vi "Teleop.vi"(10 "Match Info":T2={"Autonomous Elapsed Seconds"=0.0, "TeleOp Elapsed Seconds"=7.179, "Disabled Elapsed Seconds"=0.0, "Visited Autonomous"=FALSE, "Visited TeleOp"=TRUE, "Visited Disabled"=FALSE, "Autonomous Settings"={"Autonomous Style"=enum."Independent", "VI Refnum"=refnum}}, 11 "Call Context":T3=enum."Stop") -> ()   [LabVIEW 2020]
doc: "This VI is called for each TeleOp packet received from the DS where the robot is not disabled. It is often used to read from the joysticks and update I/O or to update setpoints for timed control loops. It should complete and return within 20 milliseconds or it may miss DS packets."
uses:
  <vilib>/Rock Robotics/WPI/DriverStation/WPI_DriverStationDerivedRobotMode.ctl
  <vilib>/Rock Robotics/WPI/DriverStation/WPI_DriverStationMatch Info.ctl
  <vilib>/Rock Robotics/WPI/ThirdParty/REV Robotics/REVLib/Typedef/Spark MAX Control Type.ctl
  <vilib>/Rock Robotics/WPI/ThirdParty/Sensors/navX/_TypeDefs/FRIC_navX_DeviceNumbersTypeDef.ctl
  <vilib>/Rock Robotics/WPI/ThirdParty/Phoenix-LabVIEW/CANCoder/Get/CTRE_Phoenix_CANcoder_GetSensorData.vi
  <vilib>/Rock Robotics/WPI/Utilities/WPI_GetSetVariantRefNum.vi
  <vilib>/addons/control/pid/pid.llb/PID (DBL).vi
  Robot Global Data.vi
  <vilib>/addons/control/pid/NI_PID_pid.lvlib
panel:
  in  "target angle":dbl=180.0
  out "MPUTemp":dbl=33.66
  in  "dt (s)":dbl=-1.0 format="%.3f"
  out "Yaw":dbl=-4.92
  in  "ScaleSpeed":dbl=0.5
  in  "PID gains 2":T1={"proportional gain (Kc)"=0.004667, "integral time (Ti, min)"=0.0, "derivative time (Td, min)"=0.0} {"derivative time (Td, min)" format="%.10f"; "integral time (Ti, min)" format="%.10f"; "proportional gain (Kc)" format="%.10f"}
  # "NOW WITH 200% MORE REV!!!!"
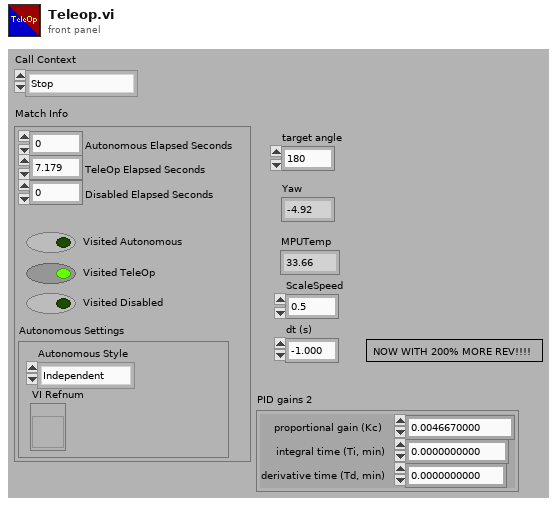
[diagram p1: front panel]
types:
  T1 = cluster{"proportional gain (Kc)":dbl, "integral time (Ti, min)":dbl, "derivative time (Td, min)":dbl}
  T2 = typedef "WPI_DriverStationMatch Info.ctl" = cluster{"Autonomous Elapsed Seconds":dbl, "TeleOp Elapsed Seconds":dbl, "Disabled Elapsed Seconds":dbl, "Visited Autonomous":bool, "Visited TeleOp":bool, "Visited Disabled":bool, "Autonomous Settings":cluster{"Autonomous Style":enum16{"Iterative", "Independent"}, "VI Refnum":refnum<vi>}}
  T3 = typedef "WPI_DriverStationDerivedRobotMode.ctl" = enum16{"Init", "Execute", "Stop"}
  T4 = typedef "FRIC_navX_DeviceNumbersTypeDef.ctl" = enum16{"Dev0", "Dev1", "Dev2", "Dev3"}
  T5 = typedef "Spark MAX Control Type.ctl" = enum16{"Percent VBus", "Voltage", "Velocity", "Position", "Smart Motion", "Current", "Smart Velocity"}
  T6 = typedef "WPI_JoystickDevRef.ctl" = cluster{"Device":T7}
  T7 = typedef "WPI_JoystickDeviceEnum.ctl" = enum16{"USB 0", "USB 1", "USB 2", "USB 3", "USB 4", "USB 5"}
  T8 = cluster{"Yaw":dbl, "Roll":dbl, "Pitch":dbl, "Heading":dbl, "Fused Heading":dbl}
  T9 = typedef "CTRE_Phoenix_CANcoder_DeviceRef.ctl" = cluster{"DeviceStatus":errorcluster, "Device Number":u8, "Handle":u64, "UsageFrame":u32, "Library Path":path}
  T10 = typedef "WPI_MotorControlDeviceRef.ctl" = cluster{"DeviceStatus":errorcluster, "Type":T11, "PWM":cluster{"PWM Channel":T12, "DeadBand":T13}, "CAN":cluster{"Device Number":u8, "SetOutput VI Ref":variant, "GetOutput VI Ref":variant, "Enable VI Ref":variant, "Disable VI Ref":variant, "Data":variant}, "Invert":bool, "DIO PWM":cluster{"PWM \"Enable\" Channel":T12, "DIOChannel":T14, "PWM Rate":dbl}}
  T11 = typedef "WPI_MotorControlType.ctl" = enum16{"PWM", "CAN", "DIO PWM"}
  T12 = typedef "FPGA_DIOPWMChannel.ctl" = enum8{"PWM 0", "PWM 1", "PWM 2", "PWM 3", "PWM 4", "PWM 5", "PWM 6", "PWM 7", "PWM 8", "PWM 9", "PWM MXP 0", "PWM MXP 1", "PWM MXP 2", "PWM MXP 3", "PWM MXP 4", "PWM MXP 5", "PWM MXP 6", "PWM MXP 7", "PWM MXP 8", "PWM MXP 9", "Invalid"}
  T13 = typedef "WPI_PWMDeadband.ctl" = cluster{"Name":string, "maxPositivePwm":i32, "minPositivePwm":i32, "centerPwm":i32, "maxNegativePwm":i32, "minNegativePwm":i32, "angularRange":u16}
  T14 = typedef "FPGA_DIOChannel.ctl" = enum8{"DIO 0", "DIO 1", "DIO 2", "DIO 3", "DIO 4", "DIO 5", "DIO 6", "DIO 7", "DIO 8", "DIO 9", "DIO MXP 0", "DIO MXP 1", "DIO MXP 2", "DIO MXP 3", "DIO MXP 4", "DIO MXP 5", "DIO MXP 6", "DIO MXP 7", "DIO MXP 8", "DIO MXP 9", "DIO MXP 10", "DIO MXP 11", "DIO MXP 12", "DIO MXP 13", "DIO MXP 14", "DIO MXP 15", "SPI Port CS1", "SPI Port CS2", "SPI Port CS3", "SPI Port MISO", "SPI Port MOSI", "Invalid"}
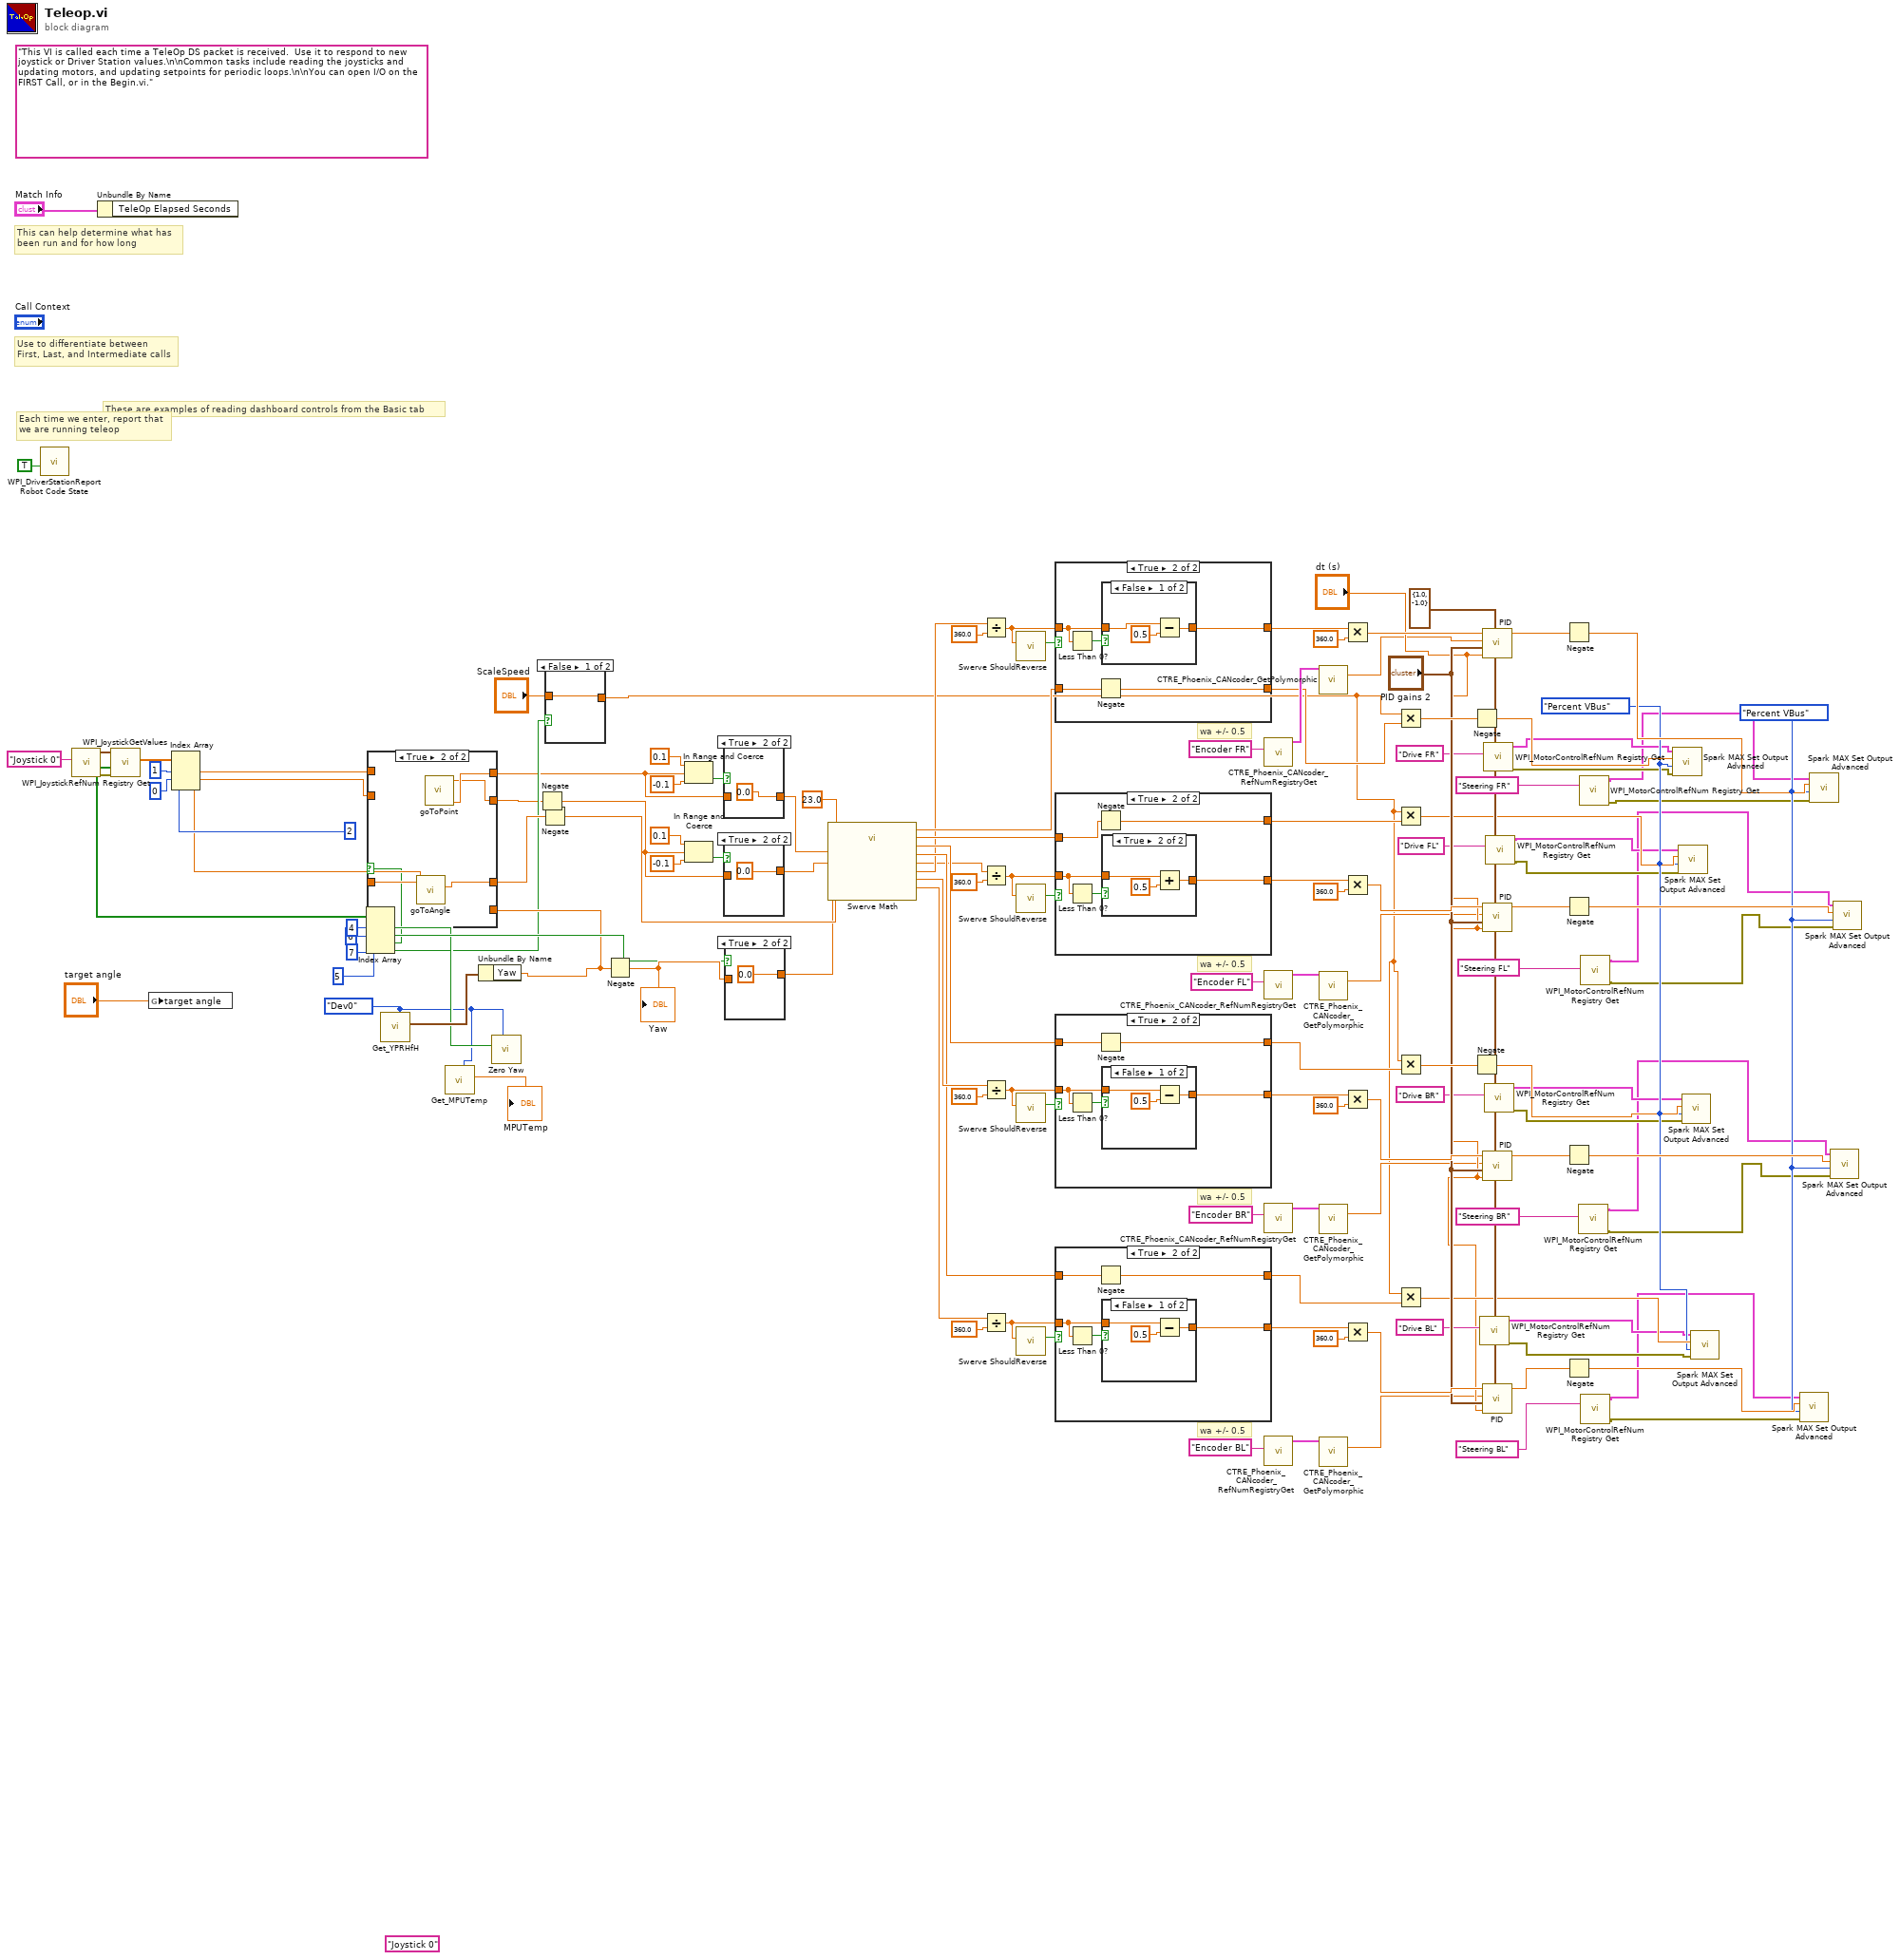
[diagram p0: block diagram]
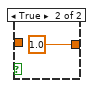
[diagram p2: hidden frame]
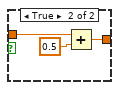
[diagram p6: hidden frame]
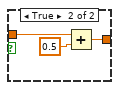
[diagram p8: hidden frame]
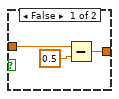
[diagram p10: hidden frame]
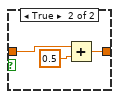
[diagram p12: hidden frame]
diagram:
  w11 = FRIC_navX_DeviceNumbersTypeDef."Dev0" ("Device Number")
  w59 = Spark_MAX_Control_Type."Percent VBus" ("Control Mode")
  w64 = Spark_MAX_Control_Type."Percent VBus" ("Control Mode")
  (unwired) "Joystick 0" ("refnum name")
  w69 = cluster{"output high":dbl, "output low":dbl} {"output high"=1.0, "output low"=-1.0} ("output range")
  w133 = 23.0 ("Trackwidth (W)")
  (unwired) "This VI is called each time a TeleOp DS packet is received.  Use it to respond to new joystick or Driver Station values.\n\nCommon tasks include reading the joysticks and updating motors, and updating setpoints for periodic loops.\n\nYou can open I/O on the FIRST Call, or in the Begin.vi."
  # "wa +/- 0.5"
  # "wa +/- 0.5"
  # "wa +/- 0.5"
  # "wa +/- 0.5"
  # "These are examples of reading dashboard controls from the Basic tab"
  # "Each time we enter, report that\nwe are running teleop"
  # "Use to differentiate between\nFirst, Last, and Intermediate calls"
  # "This can help determine what has\nbeen run and for how long"
  n1 = call <vilib>:"WPI_DriverStationReport Robot Code State.vi"("TeleOp"=TRUE ("Autonomous")) -> ()  [unwired: 10 in, 1 out]
  n2 = call <vilib>:"WPI_JoystickRefNum Registry Get.vi"("refnum name"="Joystick 0") -> ("error out"=w129:errorcluster, "JoystickDevRef"=w128:T6)  [unwired: 9 in]
  n3 = Unbundle By Name("Match Info") -> ()  [unwired: 1 out]
  n4 = call <vilib>:"WPI_JoystickGetValues.vi"("error in (no error)"=w129, "JoystickDevRef"=w128) -> ("Buttons"=w26:bool[], "Axes"=w126:dbl[])  [unwired: 5 in, 3 out]
  n5 = global write "Robot Global Data.vi" "target angle"("target angle") -> ()
  n6 = Index Array(array=w126, index #1=1 ("index"), index #2=0 ("index"), index #3=2 ("index")) -> (element #1=w3:dbl, element #2=w1:dbl, element #3=w15:dbl)
  n7 = Index Array(array=w26, index #1=4 ("index"), index #2=6 ("index"), index #3=7 ("index"), index #4=5 ("index")) -> (element #1=w13:bool, element #2=w20:bool, element #3=w5:bool, element #4=w7:bool)
  n8 = call <vilib>:"Get_YPRHfH.vi"("Device Number"=w11) -> ("YRPHfH"=w23:T8)  [unwired: 10 in]
  n9 = call <vilib>:"Get_MPUTemp.vi"("Device Number"=w11) -> ("MPUTemp"=→"MPUTemp":dbl)  [unwired: 10 in]
  n10 = Unbundle By Name(w23) -> ("Yaw"=w14:dbl)
  n11 = case shown="True" w5 {
    tunnel: [w138 w139] -> w16
    tunnel: w15 -> [w138 _]
    tunnel: w14 -> [_ _]
    tunnel: [w137 w141] -> w4
    tunnel: w3 -> [w137 _]
    tunnel: [w136 w140] -> w2
    tunnel: w1 -> [w136 _]
    frame False {
    }
    frame True {
      n12 = call "goToAngle.vi"() -> ("x2"=w139:dbl)  [unwired: 11 in]
      n13 = call "goToPoint.vi"() -> ("y result"=w141:dbl, "x result"=w140:dbl)  [unwired: 10 in]
    }
  }
  n14 = call <vilib>:"Zero Yaw.vi"("Device Number"=w11, "Zero"=w13) -> ()  [unwired: 10 in]
  n15 = Negate(x=w2) -> (-x=w28:dbl)
  n16 = Negate(x=w16) -> (-x=w27:dbl)
  n17 = case shown="False" w7 {
    tunnel: [w142 1.0 ("upper limit")] -> w9
    tunnel: "ScaleSpeed" -> [w142 _]
    frame False {
    }
    frame True {
    }
  }
  n18 = Negate(x=w14) -> (-x=w21:dbl)
  "Yaw" <- w21
  n19 = In Range and Coerce(upper limit=0.1, x=w4, lower limit=-0.1) -> (In Range?=w121:bool)  [unwired: 1 out]
  n20 = In Range and Coerce(upper limit=0.1, x=w28, lower limit=-0.1) -> (In Range?=w120:bool)  [unwired: 1 out]
  n21 = case shown="True" w121 {
    tunnel: [w144 0.0 ("upper limit")] -> w116
    tunnel: w4 -> [w144 _]
    frame False {
    }
    frame True {
    }
  }
  n22 = case shown="True" w120 {
    tunnel: [w146 0.0 ("upper limit")] -> w117
    tunnel: w28 -> [w146 _]
    frame False {
    }
    frame True {
    }
  }
  n23 = case shown="True" w20 {
    tunnel: [w148 0.0 ("upper limit")] -> w22
    tunnel: w21 -> [w148 _]
    frame False {
    }
    frame True {
    }
  }
  n24 = call "Swerve Math.vi"("Trackwidth (W)"=w133, "Wheelbase (L)"=w133, "Y -FWD"=w116, "X1 STR"=w117, "X2 RCW"=w27, "Gyro Angle in degrees"=w22) -> ("wa3"=w73:dbl, "wa4"=w71:dbl, "ws1"=w76:dbl, "ws2"=w75:dbl, "ws3"=w74:dbl, "ws4"=w72:dbl, "wa2"=w19:dbl, "wa1"=w18:dbl)  [unwired: 2 in]
  n25 = Divide(x=w19, y=360.0) -> (x/y=w113:dbl)
  n26 = Divide(x=w18, y=360.0) -> (x/y=w102:dbl)
  n27 = Divide(x=w73, y=360.0) -> (x/y=w92:dbl)
  n28 = Divide(x=w71, y=360.0) -> (x/y=w81:dbl)
  n29 = call "Swerve ShouldReverse.vi"("wa in"=w113) -> ("shouldReverse out"=w114:bool)  [unwired: 10 in]
  n30 = call "Swerve ShouldReverse.vi"("wa in"=w102) -> ("shouldReverse out"=w103:bool)  [unwired: 10 in]
  n31 = call "Swerve ShouldReverse.vi"("wa in"=w92) -> ("shouldReverse out"=w93:bool)  [unwired: 10 in]
  n32 = call "Swerve ShouldReverse.vi"("wa in"=w81) -> ("shouldReverse out"=w82:bool)  [unwired: 10 in]
  n33 = case shown="True" w114 {
    tunnel: w76 -> [w151 w152]
    tunnel: w113 -> [w150 w155]
    tunnel: [w151 w153] -> w112
    tunnel: [w150 w154] -> w111
    frame False {
    }
    frame True {
      n34 = Less Than 0?(x=w155) -> (x < 0?=w156:bool)
      n35 = Negate(x=w152) -> (-x=w153:dbl)
      n36 = case shown="False" w156 {
        tunnel: w155 -> [w158 w161]
        tunnel: [w157 w160] -> w154
        frame False {
          n37 = Subtract(x=w158, y=0.5) -> (x-y=w157:dbl)
        }
        frame True {
          n38 = Add(x=w161, y=0.5) -> (x+y=w160:dbl)
        }
      }
    }
  }
  n39 = case shown="True" w103 {
    tunnel: w75 -> [w164 w165]
    tunnel: w102 -> [w163 w168]
    tunnel: [w164 w166] -> w101
    tunnel: [w163 w167] -> w100
    frame False {
    }
    frame True {
      n40 = Less Than 0?(x=w168) -> (x < 0?=w169:bool)
      n41 = Negate(x=w165) -> (-x=w166:dbl)
      n42 = case shown="True" w169 {
        tunnel: w168 -> [w171 w174]
        tunnel: [w170 w173] -> w167
        frame False {
          n43 = Subtract(x=w171, y=0.5) -> (x-y=w170:dbl)
        }
        frame True {
          n44 = Add(x=w174, y=0.5) -> (x+y=w173:dbl)
        }
      }
    }
  }
  n45 = case shown="True" w93 {
    tunnel: w74 -> [w177 w178]
    tunnel: w92 -> [w176 w181]
    tunnel: [w177 w179] -> w91
    tunnel: [w176 w180] -> w90
    frame False {
    }
    frame True {
      n46 = Less Than 0?(x=w181) -> (x < 0?=w182:bool)
      n47 = Negate(x=w178) -> (-x=w179:dbl)
      n48 = case shown="False" w182 {
        tunnel: w181 -> [w184 w187]
        tunnel: [w183 w186] -> w180
        frame False {
          n49 = Subtract(x=w184, y=0.5) -> (x-y=w183:dbl)
        }
        frame True {
          n50 = Add(x=w187, y=0.5) -> (x+y=w186:dbl)
        }
      }
    }
  }
  n51 = case shown="True" w82 {
    tunnel: w72 -> [w190 w191]
    tunnel: w81 -> [w189 w194]
    tunnel: [w190 w192] -> w80
    tunnel: [w189 w193] -> w79
    frame False {
    }
    frame True {
      n52 = Less Than 0?(x=w194) -> (x < 0?=w195:bool)
      n53 = Negate(x=w191) -> (-x=w192:dbl)
      n54 = case shown="False" w195 {
        tunnel: w194 -> [w197 w200]
        tunnel: [w196 w199] -> w193
        frame False {
          n55 = Subtract(x=w197, y=0.5) -> (x-y=w196:dbl)
        }
        frame True {
          n56 = Add(x=w200, y=0.5) -> (x+y=w199:dbl)
        }
      }
    }
  }
  n57 = call <vilib>:"CTRE_Phoenix_CANcoder_RefNumRegistryGet.vi"("refnum name"="Encoder FR") -> ("CTRE_CANcoder_DeviceRef"=w131:T9)  [unwired: 9 in, 1 out]
  n58 = call <vilib>:"CTRE_Phoenix_CANcoder_RefNumRegistryGet.vi"("refnum name"="Encoder FL") -> ("CTRE_CANcoder_DeviceRef"=w106:T9)  [unwired: 9 in, 1 out]
  n59 = call <vilib>:"CTRE_Phoenix_CANcoder_RefNumRegistryGet.vi"("refnum name"="Encoder BR") -> ("CTRE_CANcoder_DeviceRef"=w96:T9)  [unwired: 9 in, 1 out]
  n60 = call <vilib>:"CTRE_Phoenix_CANcoder_RefNumRegistryGet.vi"("refnum name"="Encoder BL") -> ("CTRE_CANcoder_DeviceRef"=w85:T9)  [unwired: 9 in, 1 out]
  n61 = call-poly <vilib>:"CTRE_Phoenix_CANcoder_GetPolymorphic.vi"("CTRE_CANcoder_DeviceRef"=w131) -> ("Position"=w30:dbl)  [unwired: 10 in, 4 out]
  n62 = call-poly <vilib>:"CTRE_Phoenix_CANcoder_GetPolymorphic.vi"("CTRE_CANcoder_DeviceRef"=w106) -> ("Position"=w31:dbl)  [unwired: 10 in, 4 out]
  n63 = call-poly <vilib>:"CTRE_Phoenix_CANcoder_GetPolymorphic.vi"("CTRE_CANcoder_DeviceRef"=w96) -> ("Position"=w32:dbl)  [unwired: 10 in, 4 out]
  n64 = call-poly <vilib>:"CTRE_Phoenix_CANcoder_GetPolymorphic.vi"("CTRE_CANcoder_DeviceRef"=w85) -> ("Position"=w29:dbl)  [unwired: 10 in, 4 out]
  n65 = Multiply(x=w111, y=360.0) -> (x*y=w110:dbl)
  n66 = Multiply(x=w100, y=360.0) -> (x*y=w99:dbl)
  n67 = Multiply(x=w90, y=360.0) -> (x*y=w89:dbl)
  n68 = Multiply(x=w79, y=360.0) -> (x*y=w78:dbl)
  n69 = Multiply(x=w9, y=w112) -> (x*y=w108:dbl)
  n70 = Multiply(x=w9, y=w101) -> (x*y=w62:dbl)
  n71 = Multiply(x=w9, y=w91) -> (x*y=w87:dbl)
  n72 = Multiply(x=w9, y=w80) -> (x*y=w60:dbl)
  n73 = Negate(x=w108) -> (-x=w63:dbl)
  n74 = Negate(x=w87) -> (-x=w61:dbl)
  n75 = call <vilib>:"WPI_MotorControlRefNum Registry Get.vi"("refnum name"="Drive BL") -> ("error out"=w39:errorcluster, "MotorControlDevRef"=w40:T10)  [unwired: 9 in]
  n76 = call-poly <vilib>:"PID.vi"("output range"=w69, "dt (s)"="dt (s)", "PID gains"="PID gains 2", "process variable"=w30, "setpoint"=w110) -> ("output"=w132:dbl)  [unwired: 5 in, 1 out]
  n77 = call-poly <vilib>:"PID.vi"("output range"=w69, "dt (s)"="dt (s)", "PID gains"="PID gains 2", "process variable"=w31, "setpoint"=w99) -> ("output"=w107:dbl)  [unwired: 5 in, 1 out]
  n78 = call-poly <vilib>:"PID.vi"("output range"=w69, "dt (s)"="dt (s)", "PID gains"="PID gains 2", "process variable"=w32, "setpoint"=w89) -> ("output"=w97:dbl)  [unwired: 5 in, 1 out]
  n79 = call-poly <vilib>:"PID.vi"("output range"=w69, "dt (s)"="dt (s)", "PID gains"="PID gains 2", "process variable"=w29, "setpoint"=w78) -> ("output"=w86:dbl)  [unwired: 5 in, 1 out]
  n80 = call <vilib>:"WPI_MotorControlRefNum Registry Get.vi"("refnum name"="Drive FR") -> ("error out"=w56:errorcluster, "MotorControlDevRef"=w57:T10)  [unwired: 9 in]
  n81 = call <vilib>:"WPI_MotorControlRefNum Registry Get.vi"("refnum name"="Drive BR") -> ("error out"=w44:errorcluster, "MotorControlDevRef"=w45:T10)  [unwired: 9 in]
  n82 = call <vilib>:"WPI_MotorControlRefNum Registry Get.vi"("refnum name"="Drive FL") -> ("error out"=w50:errorcluster, "MotorControlDevRef"=w51:T10)  [unwired: 9 in]
  n83 = Negate(x=w132) -> (-x=w68:dbl)
  n84 = Negate(x=w107) -> (-x=w67:dbl)
  n85 = Negate(x=w97) -> (-x=w66:dbl)
  n86 = Negate(x=w86) -> (-x=w65:dbl)
  n87 = call <vilib>:"WPI_MotorControlRefNum Registry Get.vi"("refnum name"="Steering BR") -> ("error out"=w42:errorcluster, "MotorControlDevRef"=w43:T10)  [unwired: 9 in]
  n88 = call <vilib>:"WPI_MotorControlRefNum Registry Get.vi"("refnum name"="Steering FR") -> ("error out"=w53:errorcluster, "MotorControlDevRef"=w54:T10)  [unwired: 9 in]
  n89 = call <vilib>:"WPI_MotorControlRefNum Registry Get.vi"("refnum name"="Steering FL") -> ("error out"=w47:errorcluster, "MotorControlDevRef"=w48:T10)  [unwired: 9 in]
  n90 = call <vilib>:"WPI_MotorControlRefNum Registry Get.vi"("refnum name"="Steering BL") -> ("error out"=w36:errorcluster, "MotorControlDevRef"=w37:T10)  [unwired: 9 in]
  n91 = call <vilib>:"Spark MAX Set Output Advanced.vi"("error in (no error)"=w56, "Control Mode"=w59, "Setpoint"=w63, "MotorControlDevRef"=w57) -> ()  [unwired: 6 in, 2 out]
  n92 = call <vilib>:"Spark MAX Set Output Advanced.vi"("error in (no error)"=w50, "Control Mode"=w59, "Setpoint"=w62, "MotorControlDevRef"=w51) -> ()  [unwired: 6 in, 2 out]
  n93 = call <vilib>:"Spark MAX Set Output Advanced.vi"("error in (no error)"=w44, "Control Mode"=w59, "Setpoint"=w61, "MotorControlDevRef"=w45) -> ()  [unwired: 6 in, 2 out]
  n94 = call <vilib>:"Spark MAX Set Output Advanced.vi"("error in (no error)"=w39, "Control Mode"=w59, "Setpoint"=w60, "MotorControlDevRef"=w40) -> ()  [unwired: 6 in, 2 out]
  n95 = call <vilib>:"Spark MAX Set Output Advanced.vi"("error in (no error)"=w36, "Control Mode"=w64, "Setpoint"=w65, "MotorControlDevRef"=w37) -> ()  [unwired: 6 in, 2 out]
  n96 = call <vilib>:"Spark MAX Set Output Advanced.vi"("error in (no error)"=w53, "Control Mode"=w64, "Setpoint"=w68, "MotorControlDevRef"=w54) -> ()  [unwired: 6 in, 2 out]
  n97 = call <vilib>:"Spark MAX Set Output Advanced.vi"("error in (no error)"=w42, "Control Mode"=w64, "Setpoint"=w66, "MotorControlDevRef"=w43) -> ()  [unwired: 6 in, 2 out]
  n98 = call <vilib>:"Spark MAX Set Output Advanced.vi"("error in (no error)"=w47, "Control Mode"=w64, "Setpoint"=w67, "MotorControlDevRef"=w48) -> ()  [unwired: 6 in, 2 out]
